vi "Flush Data to Log File.vi"(8 "error in (no error)":errorcluster, 10 "Data Queue":T1, 11 "Logging Configuration":T2) -> (0 "error out":errorcluster)   [LabVIEW 2021, in "IMU Logging.lvlib"]
doc: "Flush the data queue of any pending data and write it to the log file. Close the TDMS file reference."
uses:
  IMU Logging.lvlib
  Logging Configuration.ctl
  Acquisition/IMU Data Queue.ctl
  IMU TimeDataStruct.ctl
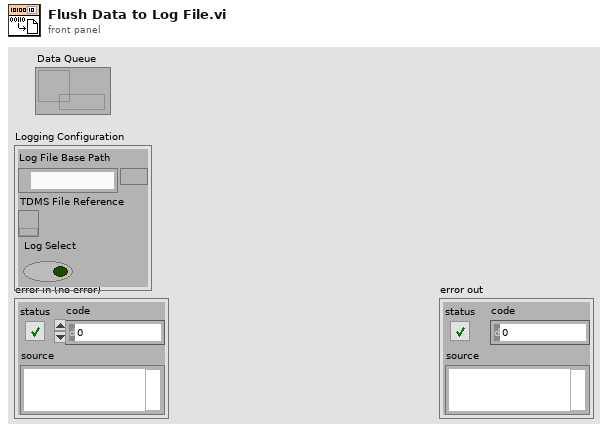
[diagram p1: front panel]
types:
  T1 = typedef "IMU Data Queue.ctl" = refnum<queue>
  T2 = typedef "IMU Logging.lvlib/Logging Configuration.ctl" = cluster{"Log File Base Path":path, "TDMS File Reference":refnum<k34>, "Log Select":bool}
  T3 = typedef "IMU TimeDataStruct.ctl" = cluster{string, dbl[]}
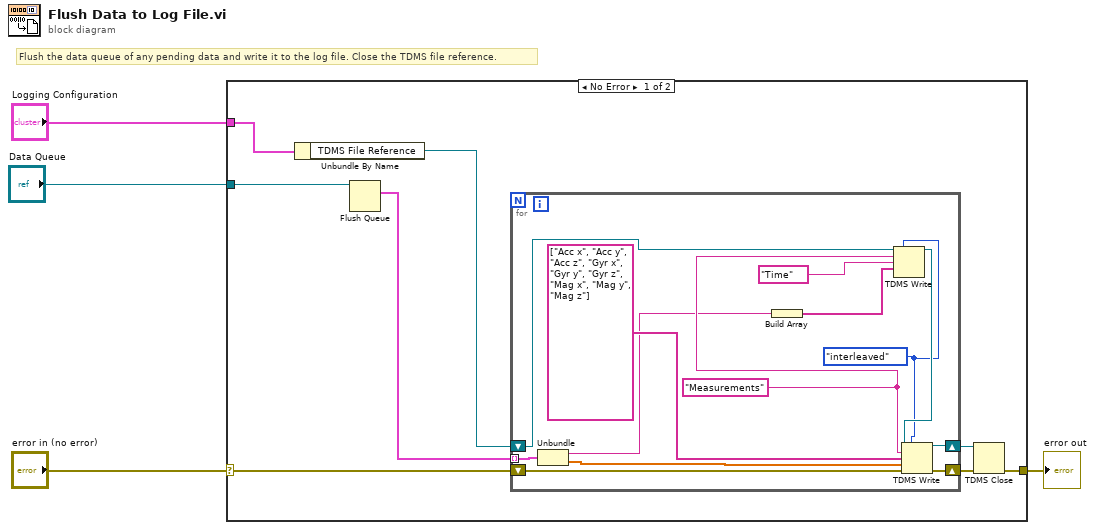
[diagram p0: block diagram]
diagram:
  # "Flush the data queue of any pending data and write it to the log file. Close the TDMS file reference."
  n1 = case shown="No Error" "error in (no error)" {
    selector: "error in (no error)" -> [w5 w26]
    tunnel: "Data Queue" -> [w8 _]
    tunnel: "Logging Configuration" -> [w7 _]
    tunnel: [w6 w26] -> w3
    frame No Error {
      n2 = Unbundle By Name(w7) -> ("TDMS File Reference"=w9:refnum<k34>)
      n3 = Flush Queue(queue=w8) -> (remaining elements=w12:T3[])  [unwired: 1 in, 2 out]
      n4 = for {
        shift-right: [w23] -> w10
        shift-left: w9 -> [w15]
        shift-right: [w24] -> w11
        shift-left: w5 -> [w25]
        tunnel: w12 -> [w22] mode=indexing
        w19 = "Measurements" ("group name in (Untitled)")
        w13 = enum16{"decimated", "interleaved"}."interleaved" ("data layout (0:decimated)")
        n5 = Unbundle(w22) -> (w18:string, w20:dbl[])
        n6 = Build Array(w18) -> (w17:string[])
        n7 = TDMS Write(0:w15, 1:w13, 5:w19, 7:"Time" ("channel name(s) in (Untitled)"), 9:w17) -> (4:w14:refnum<k34>)  [unwired: 1 in, 3 out]
        n8 = TDMS Write(0:w14, 1:w13, 5:w19, 7:string[] ["Acc x", "Acc y", "Acc z", "Gyr x", "Gyr y", "Gyr z", "Mag x", "Mag y", "Mag z"] ("channel name(s) in (Untitled)"), 9:w20, 11:w25) -> (4:w23:refnum<k34>, 15:w24:errorcluster)  [unwired: 2 out]
      }
      n9 = TDMS Close(8:w11, 11:w10) -> (0:w6:errorcluster)  [unwired: 1 out]
    }
    frame Error {
    }
  }
  "error out" <- w3
